vi "Compute Anisotropic Filter 32f.vi"(8 "Error In":errorcluster, 9 "Anisotropic Filter Parameters":T1={"Time Step"=0.1, "Total Time"=2.0, "Std. Deviation"=0.0, "Gaussian Filter X Size"=1, "Gaussian Filter Y Size"=1, "Gaussian Filter Z Size"=1} {"Gaussian Filter Z Size" min=1 max=99 step=2; "Gaussian Filter Y Size" min=1 max=99 step=2; "Gaussian Filter X Size" min=1 max=99 step=2}, 10 "Data In":sgl[][][](array[numeric]), 11 "Anisotropic Filter Object":T2={"Device In"=0, "Convolution Object"={"Device In"=0, "Program Handle"=0, "Kernel Memory Object"={"Device ID"=0, "Memeroy ID"=0, "Dimension"={"Depth"=0, "Height"=0, "Width"=0}, "Memory Type"=enum."32f"}, "Convolved Memory Object"={"Device ID"=0, "Memeroy ID"=0, "Dimension"={"Depth"=0, "Height"=0, "Width"=0}, "Memory Type"=enum."32f"}}, "Imag Kernel"=[], "Real Kernel"=[], "Convolved Buffer"={"Device ID"=0, "Memeroy ID"=0, "Dimension"={"Depth"=0, "Height"=0, "Width"=0}, "Memory Type"=enum."32f"}, "Program Handle"=0, "Ansiotropic Filter Parameters"={"Time Step"=0.0, "Total Time"=0.5, "Std. Deviation"=0.0, "Gaussian Filter X Size"=1, "Gaussian Filter Y Size"=1, "Gaussian Filter Z Size"=1}, "Raw Data"={"Device ID"=0, "Memeroy ID"=0, "Dimension"={"Depth"=0, "Height"=0, "Width"=0}, "Memory Type"=enum."32f"}, "Buffer 3"={"Device ID"=0, "Memeroy ID"=0, "Dimension"={"Depth"=0, "Height"=0, "Width"=0}, "Memory Type"=enum."32f"}, "Dimensions"={"Depth"=1, "Height"=1, "Width"=1}} {"Dimensions"."Width" min=1; "Dimensions"."Height" min=1; "Dimensions"."Depth" min=1; "Buffer 3"."Dimension"."Width" min=1; "Buffer 3"."Dimension"."Height" min=1; "Buffer 3"."Dimension"."Depth" min=1; "Raw Data"."Dimension"."Width" min=1; "Raw Data"."Dimension"."Height" min=1; "Raw Data"."Dimension"."Depth" min=1; "Ansiotropic Filter Parameters"."Gaussian Filter Z Size" min=1 max=99 step=2; "Ansiotropic Filter Parameters"."Gaussian Filter Y Size" min=1 max=99 step=2; "Ansiotropic Filter Parameters"."Gaussian Filter X Size" min=1 max=99 step=2; "Convolved Buffer"."Dimension"."Width" min=1; "Convolved Buffer"."Dimension"."Height" min=1; "Convolved Buffer"."Dimension"."Depth" min=1; "Convolution Object"."Convolved Memory Object"."Dimension"."Width" min=1; "Convolution Object"."Convolved Memory Object"."Dimension"."Height" min=1; "Convolution Object"."Convolved Memory Object"."Dimension"."Depth" min=1; "Convolution Object"."Kernel Memory Object"."Dimension"."Width" min=1; "Convolution Object"."Kernel Memory Object"."Dimension"."Height" min=1; "Convolution Object"."Kernel Memory Object"."Dimension"."Depth" min=1}) -> (0 "Error Out":errorcluster, 2 "Data Out":sgl[][][](array[numeric]), 3 "Anisotropic Filter Object Out":T2={"Device In"=0, "Convolution Object"={"Device In"=0, "Program Handle"=0, "Kernel Memory Object"={"Device ID"=0, "Memeroy ID"=0, "Dimension"={"Depth"=0, "Height"=0, "Width"=0}, "Memory Type"=enum."32f"}, "Convolved Memory Object"={"Device ID"=0, "Memeroy ID"=0, "Dimension"={"Depth"=0, "Height"=0, "Width"=0}, "Memory Type"=enum."32f"}}, "Imag Kernel"=[], "Real Kernel"=[], "Convolved Buffer"={"Device ID"=0, "Memeroy ID"=0, "Dimension"={"Depth"=0, "Height"=0, "Width"=0}, "Memory Type"=enum."32f"}, "Program Handle"=0, "Ansiotropic Filter Parameters"={"Time Step"=0.0, "Total Time"=0.5, "Std. Deviation"=0.0, "Gaussian Filter X Size"=1, "Gaussian Filter Y Size"=1, "Gaussian Filter Z Size"=1}, "Raw Data"={"Device ID"=0, "Memeroy ID"=0, "Dimension"={"Depth"=0, "Height"=0, "Width"=0}, "Memory Type"=enum."32f"}, "Buffer 3"={"Device ID"=0, "Memeroy ID"=0, "Dimension"={"Depth"=0, "Height"=0, "Width"=0}, "Memory Type"=enum."32f"}, "Dimensions"={"Depth"=1, "Height"=1, "Width"=1}} {"Dimensions"."Width" min=1; "Dimensions"."Height" min=1; "Dimensions"."Depth" min=1; "Buffer 3"."Dimension"."Width" min=1; "Buffer 3"."Dimension"."Height" min=1; "Buffer 3"."Dimension"."Depth" min=1; "Raw Data"."Dimension"."Width" min=1; "Raw Data"."Dimension"."Height" min=1; "Raw Data"."Dimension"."Depth" min=1; "Ansiotropic Filter Parameters"."Gaussian Filter Z Size" min=1 max=99 step=2; "Ansiotropic Filter Parameters"."Gaussian Filter Y Size" min=1 max=99 step=2; "Ansiotropic Filter Parameters"."Gaussian Filter X Size" min=1 max=99 step=2; "Convolved Buffer"."Dimension"."Width" min=1; "Convolved Buffer"."Dimension"."Height" min=1; "Convolved Buffer"."Dimension"."Depth" min=1; "Convolution Object"."Convolved Memory Object"."Dimension"."Width" min=1; "Convolution Object"."Convolved Memory Object"."Dimension"."Height" min=1; "Convolution Object"."Convolved Memory Object"."Dimension"."Depth" min=1; "Convolution Object"."Kernel Memory Object"."Dimension"."Width" min=1; "Convolution Object"."Kernel Memory Object"."Dimension"."Height" min=1; "Convolution Object"."Kernel Memory Object"."Dimension"."Depth" min=1}, 4 "Time in ms":dbl)   [LabVIEW 2012, in "OpenCLV x64.lvlib"]
uses:
  OpenCLV x64.lvlib
  Controls/Anisotropic Filter Object.ctl
  Controls/Device ID.ctl
  Controls/Convolution Object.ctl
  Controls/Program Handle.ctl
  Controls/Memory Object.ctl
  Controls/Memory ID.ctl
  User Controls/Array Dimensions.ctl
  Controls/Memory Type.ctl
  Controls/Anisotropic Filter Parameters.ctl
  Write Memory/WriteMemory_32f.vi
  Read Memory/ReadMemory_32f.vi
  Set Kernel Arguments/Set Kernel Arguments Memory Object.vi
  Set Kernel Arguments/Set Kernel Arguments 32f.vi
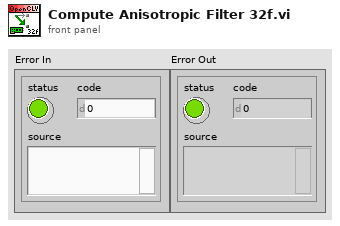
[diagram p1: front panel]
types:
  T1 = typedef "OpenCLV x64.lvlib/Anisotropic Filter Parameters.ctl" = cluster{"Time Step":sgl, "Total Time":sgl, "Std. Deviation":sgl, "Gaussian Filter X Size":u32, "Gaussian Filter Y Size":u32, "Gaussian Filter Z Size":u32}
  T2 = typedef "OpenCLV x64.lvlib/Anisotropic Filter Object.ctl" = cluster{"Device In":T3, "Convolution Object":T4, "Imag Kernel":sgl[][][], "Real Kernel":sgl[][][], "Convolved Buffer":T6, "Program Handle":T5, "Ansiotropic Filter Parameters":T1, "Raw Data":T6, "Buffer 3":T6, "Dimensions":T8}
  T3 = typedef "OpenCLV x64.lvlib/Device ID.ctl" = u64
  T4 = typedef "OpenCLV x64.lvlib/Convolution Object.ctl" = cluster{"Device In":T3, "Program Handle":T5, "Kernel Memory Object":T6, "Convolved Memory Object":T6}
  T5 = typedef "OpenCLV x64.lvlib/Program Handle.ctl" = u64
  T6 = typedef "OpenCLV x64.lvlib/Memory Object.ctl" = cluster{"Device ID":T3, "Memeroy ID":T7, "Dimension":T8, "Memory Type":T9}
  T7 = typedef "OpenCLV x64.lvlib/Memory ID.ctl" = u64
  T8 = typedef "Array Dimensions.ctl" = cluster{"Depth":u64, "Height":u64, "Width":u64}
  T9 = typedef "OpenCLV x64.lvlib/Memory Type.ctl" = enum16{"32f", "u8", "i8", "u16", "i16", "u32", "i32", "64f"}
  T10 = typedef "OpenCLV x64.lvlib/Kernel Handle.ctl" = u64
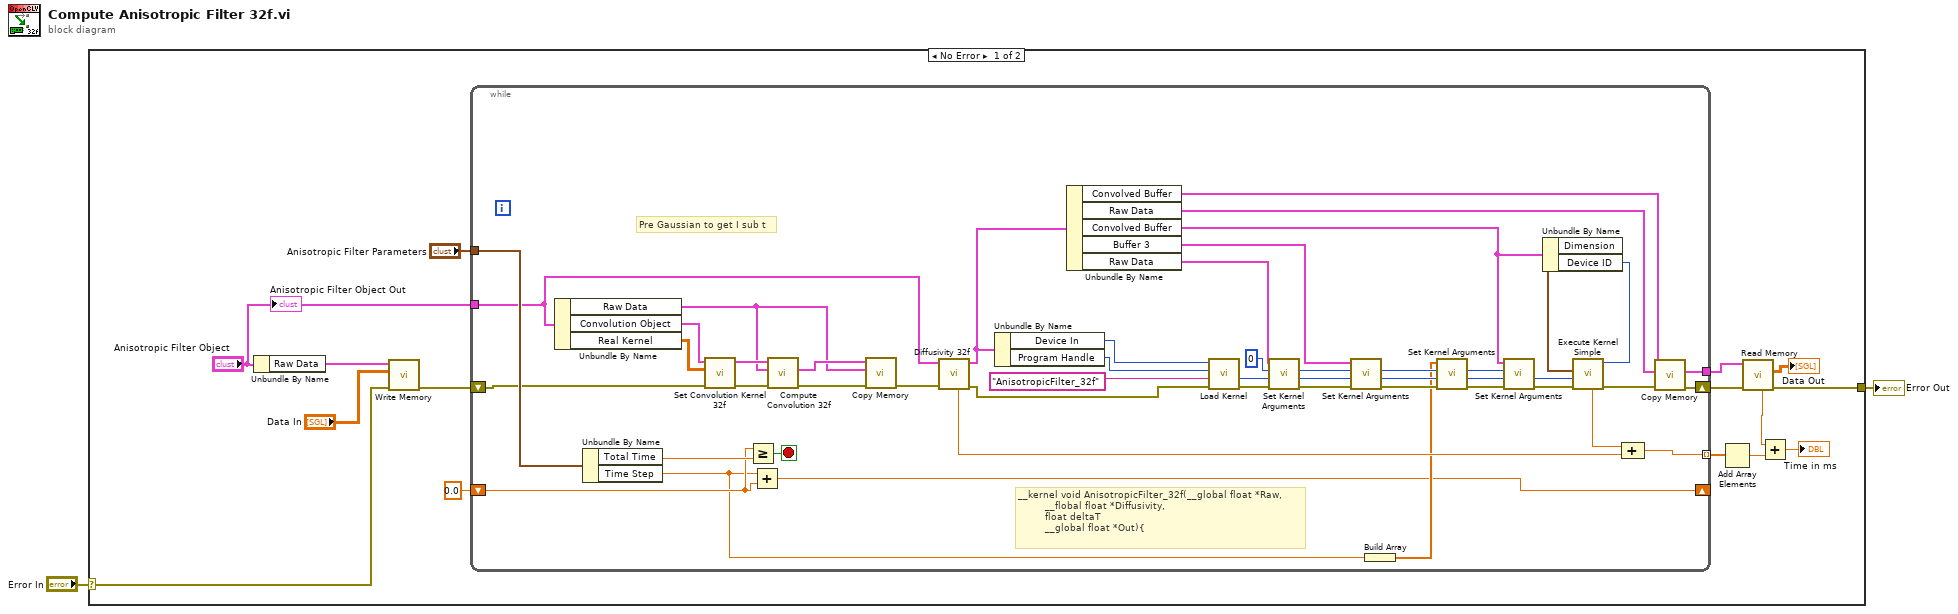
[diagram p0: block diagram]
diagram:
  n1 = case shown="No Error" "Error In" {
    selector: "Error In" -> [w8 w67]
    tunnel: [w15 w67] -> w1
    frame No Error {
      n2 = Unbundle By Name("Anisotropic Filter Object") -> ("Raw Data"=w7:T6)
      n3 = call-poly "Write Memory.vi"("Error In"=w8, "Data In"="Data In", "Memory Object In"=w7) -> ("Error Out"=w10:errorcluster)  [unwired: 6 in, 2 out]
      n4 = while {
        tunnel: "Anisotropic Filter Object" -> [w27]
        shift-right: [w45] -> w17
        shift-left: w10 -> [w30]
        tunnel: [w44] -> w16
        tunnel: [w46] -> w14 mode=indexing
        shift-right: [w22] -> _
        shift-left: sgl 0.0 -> [w19]
        tunnel: "Anisotropic Filter Parameters" -> [w34]
        stop <- w20 stop-if-true
        # "Pre Gaussian to get I sub t"
        # "__kernel void AnisotropicFilter_32f(__global float *Raw,\n\t\t\t\t\t\t\t\t\t__flobal float *Diffusivity,\n\t\t\t\t\t\t\t\t\tfloat deltaT\n\t\t\t\t\t\t\t\t\t__global float *Out){"
        n5 = Unbundle By Name(w27) -> ("Raw Data"=w23:T6, "Convolution Object"=w24:T4, "Real Kernel"=w31:sgl[][][])
        n6 = Unbundle By Name(w34) -> ("Total Time"=w21:sgl, "Time Step"=w18:sgl)
        n7 = call "Set Convolution Kernel 32f.vi"("Error In"=w30, "Kernel In"=w31, "Convolution Object"=w24) -> ("Error Out"=w32:errorcluster, "Convolution Object Out"=w25:T4)  [unwired: 7 in]
        n8 = Greater Or Equal?(x=w19, y=w21) -> (x >= y?=w20:bool)
        n9 = Add(x=w18, y=w19) -> (x+y=w22:sgl)
        n10 = call "Compute Convolution 32f.vi"("Error In"=w32, "Input Memory"=w23, "Convolution Object"=w25) -> ("Error Out"=w29:errorcluster, "Convolved Memory"=w26:T6)  [unwired: 5 in, 2 out]
        n11 = call "Copy Memory.vi"("Error In"=w29, "Destination Object"=w23, "Source Object"=w26) -> ("Error Out"=w28:errorcluster)  [unwired: 6 in, 2 out]
        n12 = call "Diffusivity 32f.vi"("Error In"=w28, "Anisotropic Filter Object"=w27) -> ("Error Out"=w42:errorcluster, "Anisotropic Filter Object Out"=w65:T2, "Time in ms"=w66:dbl)  [unwired: 7 in]
        n13 = Unbundle By Name(w65) -> ("Device In"=w64:T3, "Program Handle"=w63:T5)
        n14 = Unbundle By Name(w65) -> ("Convolved Buffer"=w39:T6, "Raw Data"=w43:T6, "Convolved Buffer"=w40:T6, "Buffer 3"=w36:T6, "Raw Data"=w61:T6)
        n15 = call "Load Kernel.vi"("Error In"=w42, "Kernel Name"="AnisotropicFilter_32f", "Program Handle"=w63, "Device In"=w64) -> ("Error Out"=w59:errorcluster, "Kernel Handle"=w60:T10)  [unwired: 4 in, 2 out]
        n16 = call-poly "Set Kernel Arguments.vi"("Error In"=w59, "Kernel Handle"=w60, "Argument Number"=0, "Memory Object"=w61) -> ("Error Out"=w57:errorcluster, "Kernel Handle out"=w56:T10, "Auto Inc Arugment Number"=w55:i32)  [unwired: 5 in]
        n17 = call-poly "Set Kernel Arguments.vi"("Error In"=w57, "Kernel Handle"=w56, "Argument Number"=w55, "Memory Object"=w36) -> ("Error Out"=w54:errorcluster, "Kernel Handle out"=w53:T10, "Auto Inc Arugment Number"=w52:i32)  [unwired: 5 in]
        n18 = Build Array(w18) -> (w33:sgl[])
        n19 = call-poly "Set Kernel Arguments.vi"("Error In"=w54, "Kernel Handle"=w53, "Argument Number"=w52, "32f Constant"=w33) -> ("Error Out"=w50:errorcluster, "Kernel Handle out"=w51:T10, "Auto Inc Arugment Number"=w49:i32)  [unwired: 5 in]
        n20 = call-poly "Set Kernel Arguments.vi"("Error In"=w50, "Kernel Handle"=w51, "Argument Number"=w49, "Memory Object"=w40) -> ("Error Out"=w35:errorcluster, "Kernel Handle out"=w37:T10)  [unwired: 5 in, 1 out]
        n21 = Unbundle By Name(w40) -> ("Dimension"=w41:T8, "Device ID"=w48:T3)
        n22 = call "Execute Kernel Simple.vi"("Error In"=w35, "Kernel Handle"=w37, "Thread Dimensions"=w41, "Device In"=w48) -> ("Error Out"=w38:errorcluster, "Time in ms"=w47:dbl)  [unwired: 4 in, 2 out]
        n23 = Compound Arithmetic op=ADD(w47, w66) -> (w46:dbl)
        n24 = call "Copy Memory.vi"("Error In"=w38, "Destination Object"=w43, "Source Object"=w39) -> ("Error Out"=w45:errorcluster, "Destination Object Out"=w44:T6)  [unwired: 6 in, 1 out]
      }
      n25 = Add Array Elements(numeric array=w14) -> (sum=w13:dbl)
      n26 = call-poly "Read Memory.vi"("Error In"=w17, "Memory Object In"=w16) -> ("Error Out"=w15:errorcluster, "Data Out"=→"Data Out":sgl[][][], "ms"=w12:dbl)  [unwired: 6 in, 1 out]
      n27 = Add(x=w12, y=w13) -> (x+y=→"Time in ms":dbl)
      "Anisotropic Filter Object Out" <- "Anisotropic Filter Object"
    }
    frame Error {
    }
  }
  "Error Out" <- w1
